vi "ExcuseNote_Panel.vi"(8 "error in (no error)":errorcluster, 11 "PanelController":refnum<class "MemberPanel.lvclass">) -> (0 "error out":errorcluster, 3 "Member_Actor.lvlib:ExcuseNote.lvclass":refnum<class "ExcuseNote.lvclass">)   [LabVIEW 2015, in "Member_Actor.lvlib"]
uses:
  Member_Actor.lvlib
  ExcuseNote/ExcuseNote.lvclass
  MemberPanel/MemberPanel.lvclass
  <vilib>/Utility/error.llb/Error Cluster From Error Code.vi
  <vilib>/ErrorRing/Error Ring.xnode
panel:
  in  "ExcuseNote":T1
  in  "提交":bool
  in  "Stop":bool
  # "(*如果只请假了一节课，重复填写即可)"
  # "-"
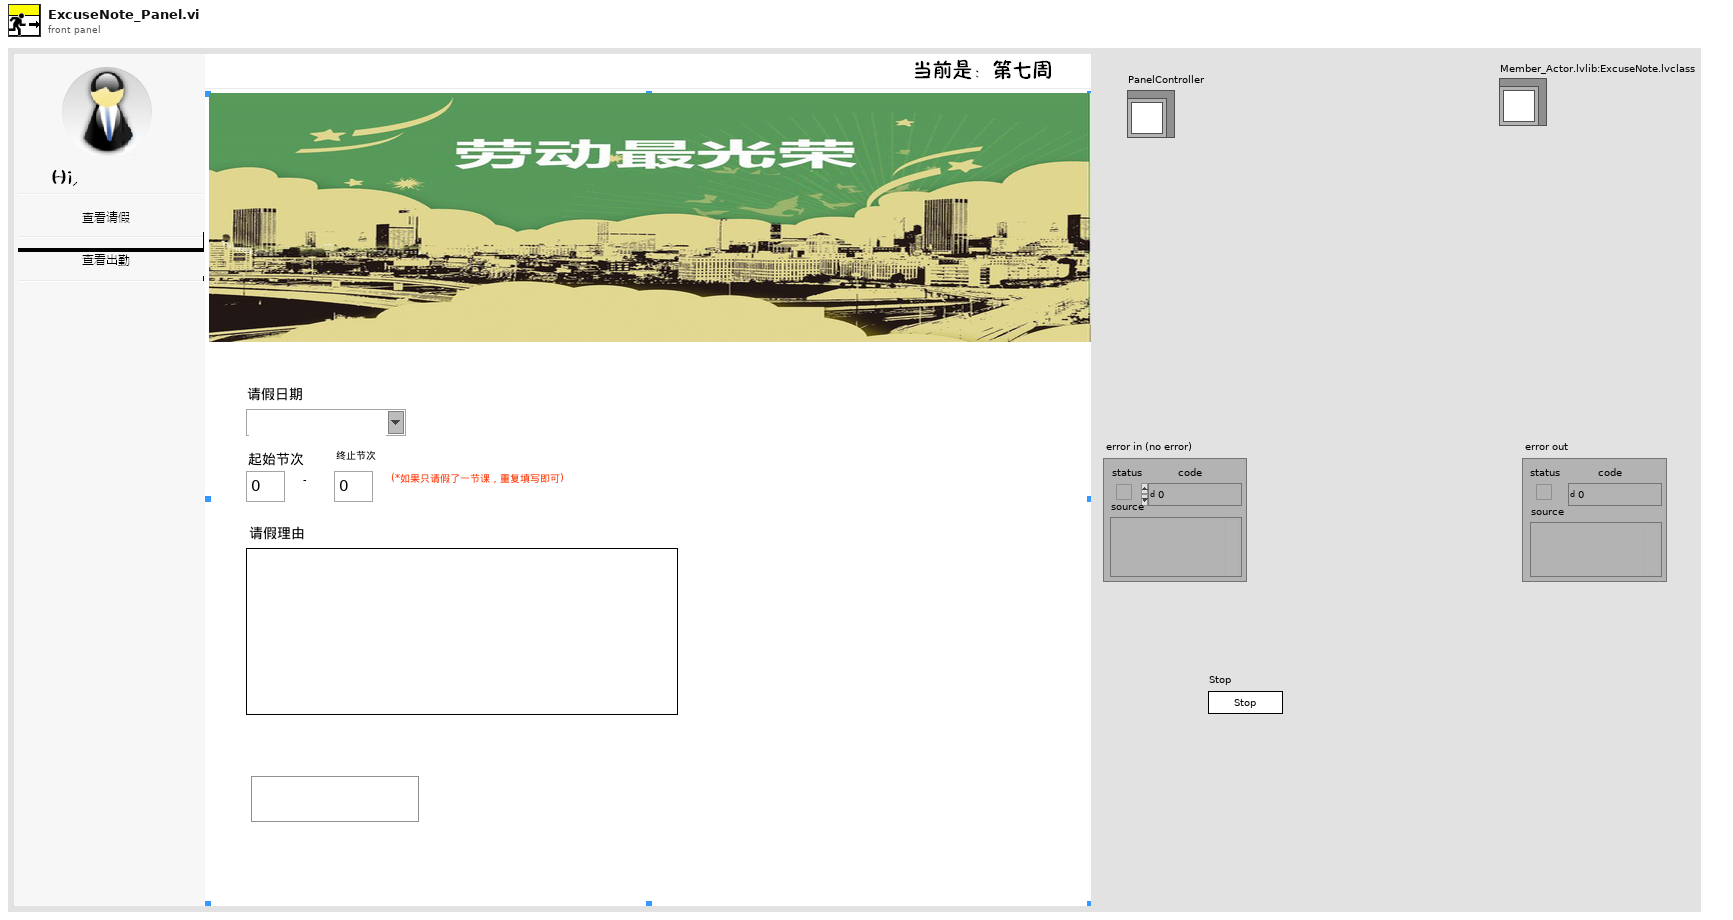
[diagram p1: front panel]
types:
  T1 = cluster{"请假日期":string, "起始节次":i32, "终止节次":i32, "请假理由":string}
  T2 = enum32{"Invalid", "Standard", "Closed", "Hidden", "Minimized", "Maximized"}
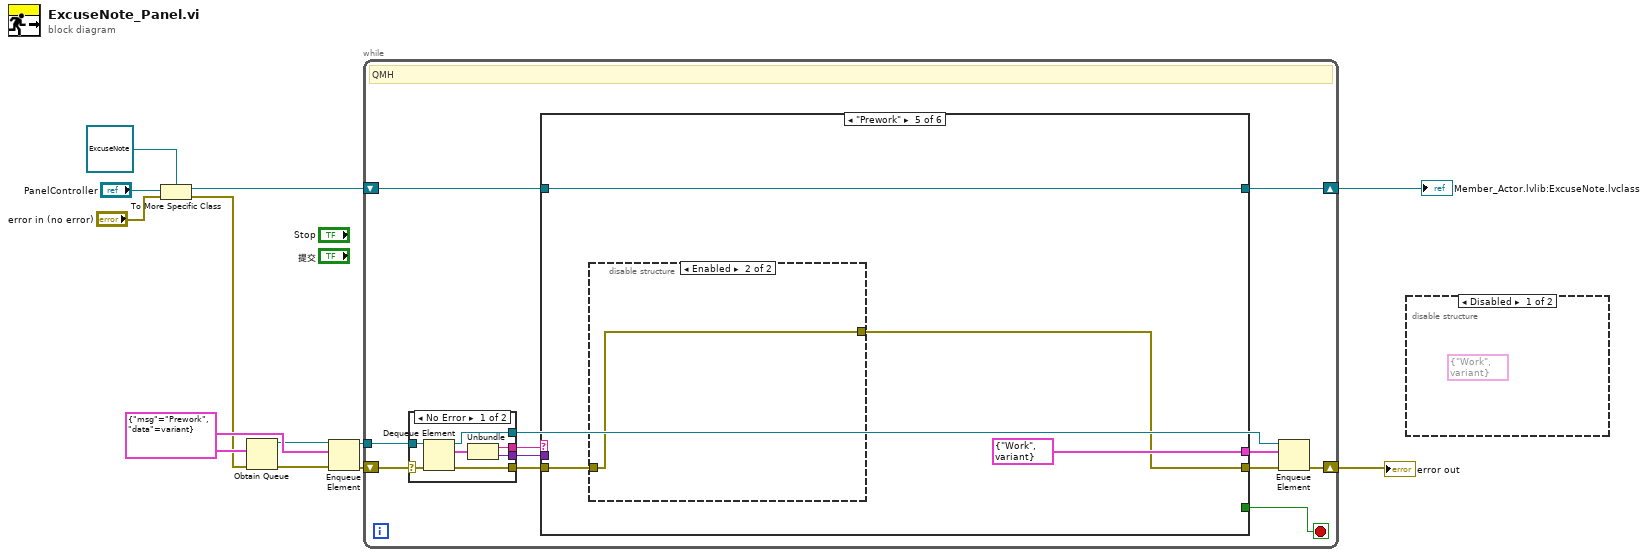
[diagram p0: block diagram]
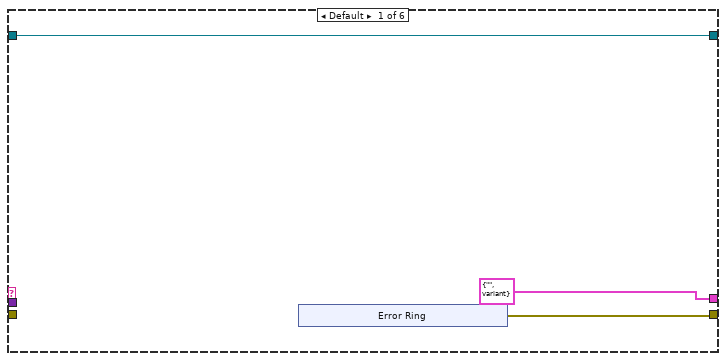
[diagram p3: hidden frame]
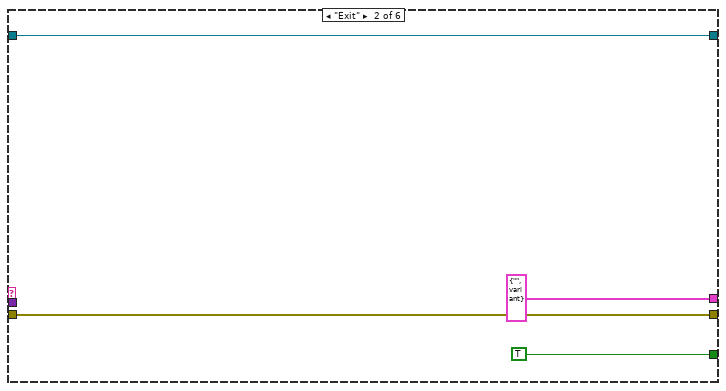
[diagram p4: hidden frame]
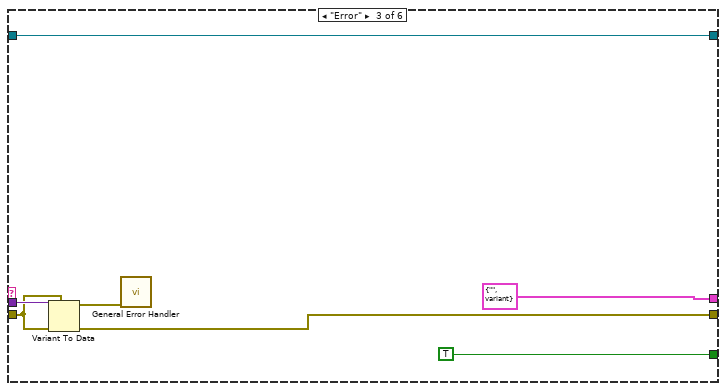
[diagram p5: hidden frame]
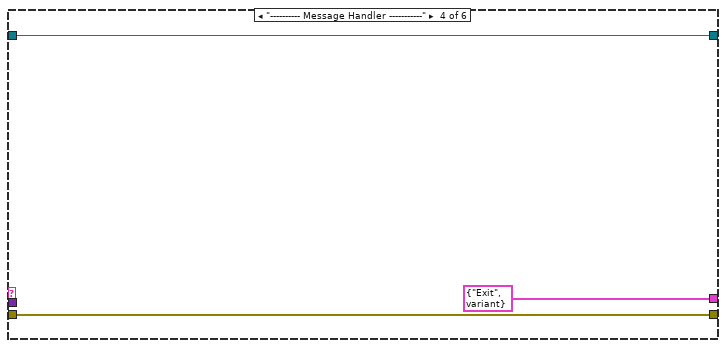
[diagram p6: hidden frame]
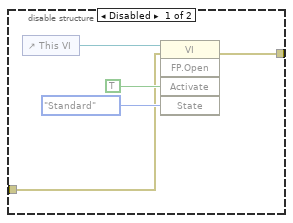
[diagram p7: hidden frame]
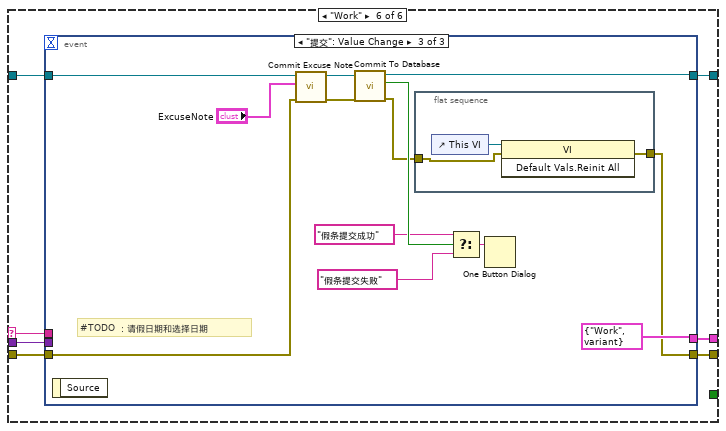
[diagram p8: hidden frame]
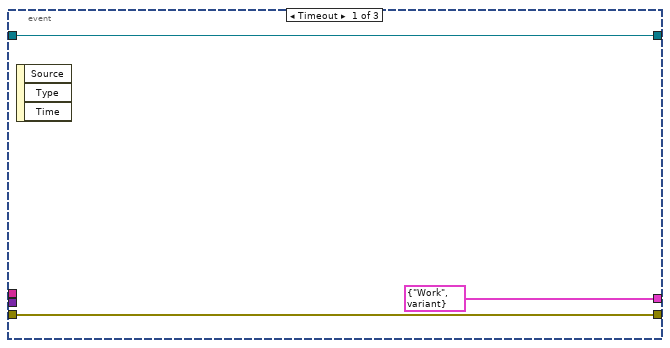
[diagram p9: hidden frame]
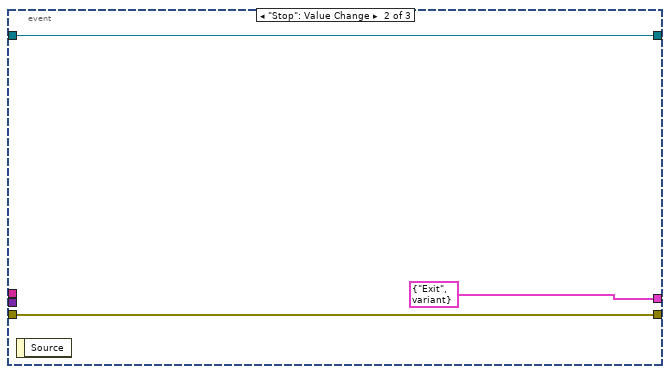
[diagram p10: hidden frame]
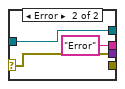
[diagram p11: hidden frame]
diagram:
  w10 = cluster{"msg":string, "data":variant} {"msg"="Prework", "data"=variant}
  n1 = To More Specific Class(target class=refnum<class "ExcuseNote.lvclass"> refnum ("PanelController"), reference="PanelController", error in="error in (no error)") -> (specific class reference=w4:refnum<class "ExcuseNote.lvclass">, error out=w2:errorcluster)
  n2 = Obtain Queue(element data type=w10, error in (no error)=w2) -> (queue out=w8:refnum<queue>, error out=w9:errorcluster)  [unwired: 3 in, 1 out]
  n3 = Enqueue Element(queue=w8, element=w10, error in (no error)=w9) -> (queue out=w11:refnum<queue>, error out=w12:errorcluster)  [unwired: 1 in, 1 out]
  n4 = while {
    tunnel: w11 -> [w23]
    shift-right: [w18] -> w1
    shift-left: w12 -> [w24]
    shift-right: [w13] -> w7
    shift-left: w4 -> [w14]
    stop <- w15 stop-if-true
    # "QMH"
    n5 = case shown="No Error" w24 {
      selector: w24 -> [w91 w95]
      tunnel: w23 -> [w92 w93]
      tunnel: [w90 _] -> w22
      tunnel: [w88 "Error" ("msg")] -> w21
      tunnel: [w87 w95] -> w20
      tunnel: [w86 w93] -> w17
      frame No Error {
        n6 = Dequeue Element(queue=w92, error in (no error)=w91) -> (queue out=w86:refnum<queue>, element=w89:cluster{"msg":string, "data":variant}, error out=w90:errorcluster)  [unwired: 1 in, 1 out]
        n7 = Unbundle(w89) -> ("msg"=w88:string, "data"=w87:variant)
      }
      frame Error {
      }
    }
    n8 = case shown="\"Prework\"" w21 {
      selector: w21 -> [_ _ _ _ _ w61]
      tunnel: w22 -> [_ w36 w42 w46 w48 w63]
      tunnel: w20 -> [_ _ w43 _ _ w62]
      tunnel: [w27 w36 w40 w46 w47 w60] -> w19
      tunnel: [cluster{"msg":string, "data":variant} {"msg"="", "data"=variant} cluster{"msg":string, "data":variant} {"msg"="", "data"=variant} cluster{"msg":string, "data":variant} {"msg"="", "data"=variant} cluster{"msg":string, "data":variant} {"msg"="Exit", "data"=variant} cluster{"msg":string, "data":variant} {"msg"="Work", "data"=variant} w59] -> w16
      tunnel: [_ TRUE TRUE _ _ _] -> w15
      tunnel: w14 -> [w25 w33 w37 w44 w49 w58]
      tunnel: [w25 w33 w37 w44 w49 w57] -> w13
      frame Default {
        n9 = xnode "Error Ring"() -> ("error out"=w27:errorcluster)
      }
      frame "Exit" {
      }
      frame "Error" {
        n10 = Variant To Data(error in=w42, type=w42, Variant=w43) -> (data=w41:errorcluster, error out=w40:errorcluster)
        n11 = call <vilib>:"General Error Handler.vi"("error in (no error)"=w41) -> ()  [unwired: 10 in, 5 out]
      }
      frame "---------- Message Handler -----------" {
      }
      frame "Prework" {
        n12 = disable-structure shown="Enabled" {
          disable-tunnel: w48 -> [w52 w56]
          disable-tunnel: [w51 w56] -> w47
          frame Disabled {
            n13 = control-ref of="This VI"() -> (w55:refnum<vi>)
            n14 = invoke class="VI" method="FP.Open"(reference=w55, error in=w52, "Activate"=TRUE ("Activate?"), "State"=T2."Standard") -> (error out=w51:errorcluster)  [unwired: 1 in, 4 out]
          }
          frame Enabled {
          }
        }
      }
      frame "Work" {
        n15 = event shown="[2] \"提交\": Value Change" {
          selector: _ -> [_ _ _]
          dyn-events: _ -> [_ _ _]
          timeout: _ -> [_ _ _]
          tunnel: w63 -> [w66 w69 w81]
          tunnel: w62 -> [_ _ _]
          tunnel: w61 -> [_ _ _]
          tunnel: [w66 w69 w71] -> w60
          tunnel: [cluster{"msg":string, "data":variant} {"msg"="Work", "data"=variant} cluster{"msg":string, "data":variant} {"msg"="Exit", "data"=variant} cluster{"msg":string, "data":variant} {"msg"="Work", "data"=variant}] -> w59
          tunnel: w58 -> [w64 w67 w82]
          tunnel: [w64 w67 w77] -> w57
          event Timeout {
            n16 = event-data() -> ()  [unwired: 1 in, 3 out]
          }
          event "Stop": Value Change {
            n17 = event-data() -> ()  [unwired: 1 in, 1 out]
          }
          event "提交": Value Change {
            # "#TODO ：请假日期和选择日期"
            n18 = event-data() -> ()  [unwired: 1 in, 1 out]
            n19 = call "Commit Excuse Note.vi"("error in (no error)"=w81, "ExcuseNote"="ExcuseNote", "ExcuseNote in"=w82) -> ("error out"=w78:errorcluster, "ExcuseNote out"=w79:refnum<class "ExcuseNote.lvclass">)  [unwired: 7 in]
            n20 = call "Commit To Database.vi"("error in (no error)"=w78, "ExcuseNote in"=w79) -> ("error out"=w72:errorcluster, "CommitSuccess(True)"=w76:bool, "ExcuseNote out"=w77:refnum<class "ExcuseNote.lvclass">)  [unwired: 7 in]
            n21 = flat-sequence {
              tunnel: w72 -> [w84]
              tunnel: [w83] -> w71
              frame #0 {
                n22 = control-ref of="This VI"() -> (w85:refnum<vi>)
                n23 = invoke class="VI" method="Default Vals.Reinit All"(reference=w85, error in=w84) -> (error out=w83:errorcluster)  [unwired: 1 in, 2 out]
              }
            }
            n24 = Select(t="假条提交成功", s=w76, f="假条提交失败") -> (s? t:f=w73:string)
            n25 = One Button Dialog(message=w73) -> ()  [unwired: 1 in, 1 out]
          }
        }
      }
    }
    n26 = Enqueue Element(queue=w17, element=w16, error in (no error)=w19) -> (error out=w18:errorcluster)  [unwired: 1 in, 2 out]
  }
  "Member_Actor.lvlib:ExcuseNote.lvclass" <- w7
  "error out" <- w1
  n27 = disable-structure shown="Disabled" {
    frame Disabled {
      (unwired) cluster{"msg":string, "data":variant} {"msg"="Work", "data"=variant}
    }
    frame Enabled {
    }
  }
